vi "Memory Cell to bool.vi"(7 "Field Selector":T1, 10 "Memory Cell":T2={"type"=enum."float", "x"=0.0, "y"=0.0, "z"=0.0, "w"=0.0}) -> (2 "bool out":bool)   [LabVIEW 2017]
uses:
  Type Definitions/Memory Cell.ctl
  Type Definitions/Memory Cell Type Enum.ctl
  Type Definitions/Cell Selector.ctl
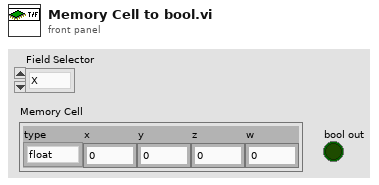
[diagram p1: front panel]
types:
  T1 = typedef "Cell Selector.ctl" = enum16{"X", "Y", "Z", "W"}
  T2 = typedef "Memory Cell.ctl" = cluster{"type":T3, "x":dbl, "y":dbl, "z":dbl, "w":dbl}
  T3 = typedef "Memory Cell Type Enum.ctl" = enum16{"integer", "float", "vector", "rotation"}
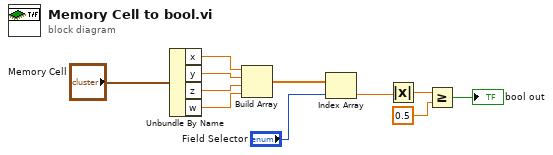
[diagram p0: block diagram]
diagram:
  n1 = Unbundle By Name("Memory Cell") -> ("x"=w10:dbl, "y"=w9:dbl, "z"=w8:dbl, "w"=w7:dbl)
  n2 = Build Array(w10, w9, w8, w7) -> (w6:dbl[])
  n3 = Index Array(array=w6, index="Field Selector") -> (element=w4:dbl)
  n4 = Absolute Value(x=w4) -> (abs(x)=w3:dbl)
  n5 = Greater Or Equal?(x=w3, y=0.5) -> (x >= y?=→"bool out":bool)
